vi "PLC_Trigger_Gen.vi"(5 "0_Stop":bool, 6 "Product Code":string, 7 "Station Number":string, 10 "Trig":bool[](array[boolean]), 11 "Trig old":bool[](array[boolean])) -> (3 "State to Log":T1(array[cluster]))   [LabVIEW 2017]
panel:
  in  "Ack old":bool[](array[boolean])
  in  "Ack":bool[](array[boolean])
  in  "Station No":u32
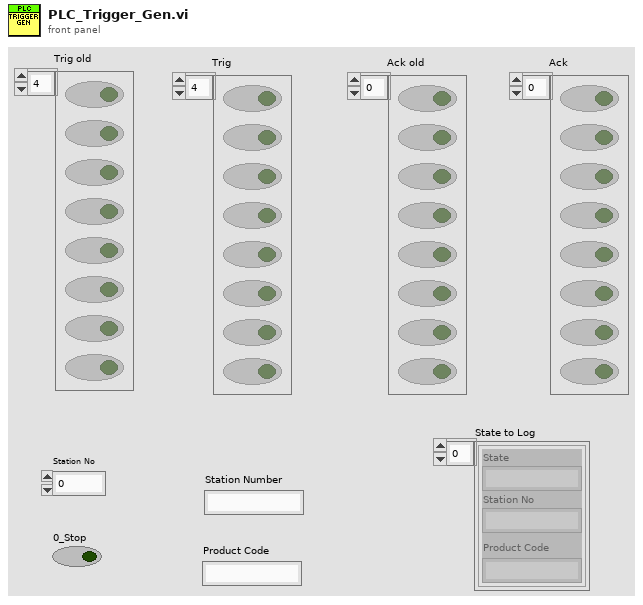
[diagram p1: front panel]
types:
  T1 = cluster{"State":string, "Station No":string, "Product Code":string}[]
  T2 = cluster{"State":string, "Station No":string, "Product Code":string}
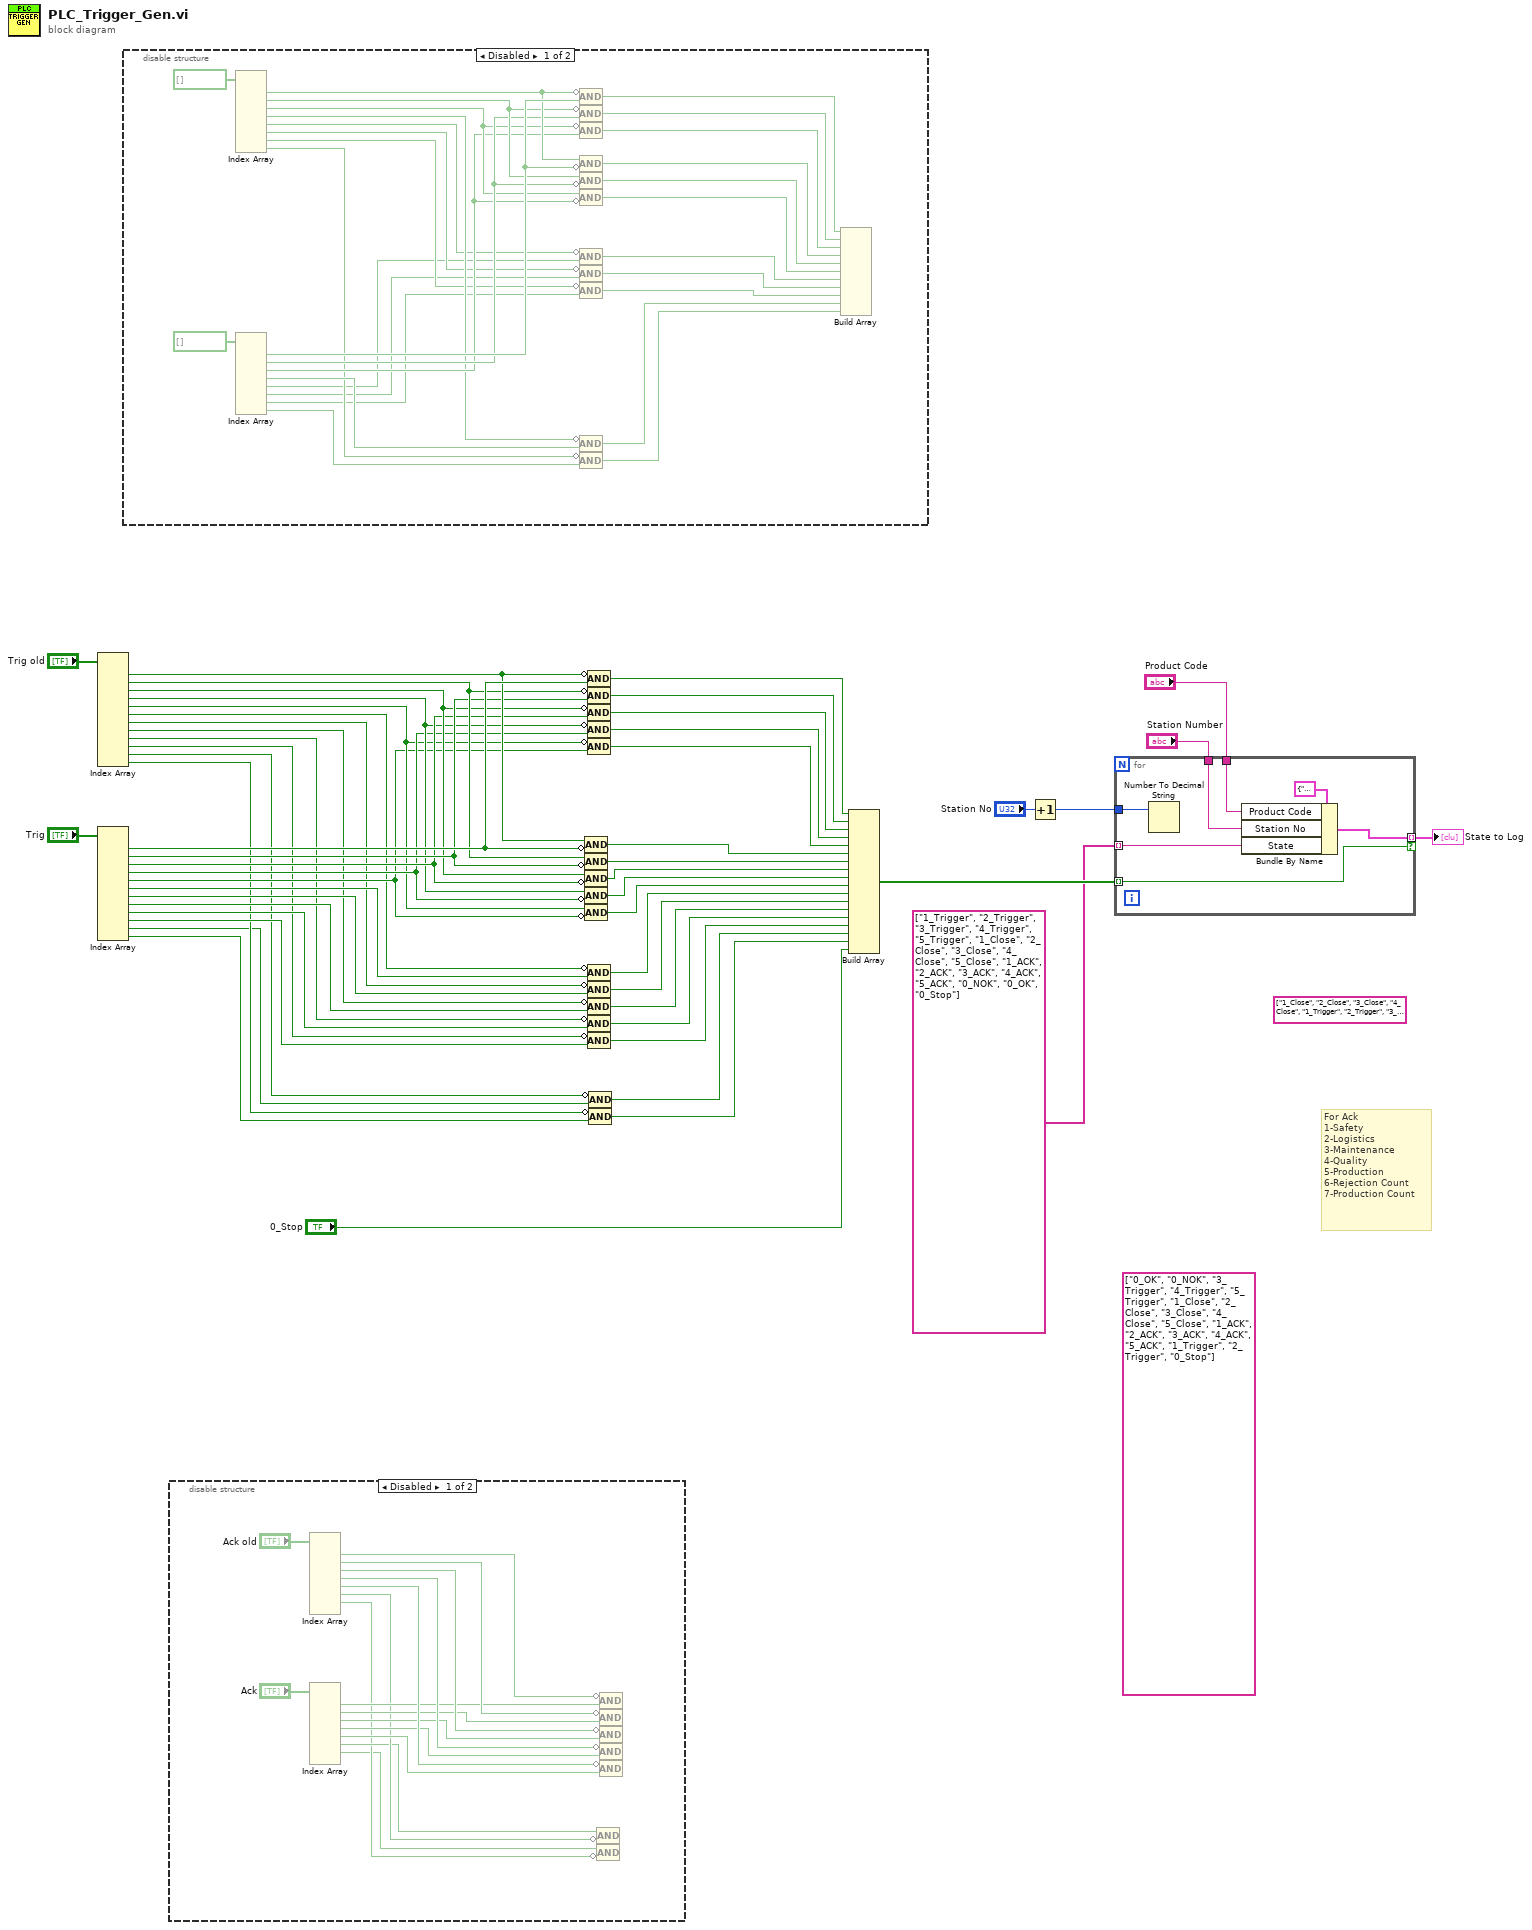
[diagram p0: block diagram]
diagram:
  (unwired) string[] ["1_Close", "2_Close", "3_Close", "4_Close", "1_Trigger", "2_Trigger", "3_Trigger", "4_Trigger", "1_ACK", "2_ACK", "3_ACK", "4_ACK", "0_Stop", "0_OK", "0_NOK"]
  (unwired) string[] ["0_OK", "0_NOK", "3_Trigger", "4_Trigger", "5_Trigger", "1_Close", "2_Close", "3_Close", "4_Close", "5_Close", "1_ACK", "2_ACK", "3_ACK", "4_ACK", "5_ACK", "1_Trigger", "2_Trigger", "0_Stop"]
  # "For Ack\n1-Safety\n2-Logistics\n3-Maintenance\n4-Quality\n5-Production\n6-Rejection Count\n7-Production Count"
  n1 = Index Array(array="Trig old") -> (element #1=w48:bool, element #2=w47:bool, element #3=w45:bool, element #4=w43:bool, element #5=w41:bool, element #6=w22:bool, element #7=w20:bool, element #8=w18:bool, element #9=w16:bool, element #10=w14:bool, element #11=w12:bool, element #12=w11:bool)  [unwired: 12 in]
  n2 = Index Array(array="Trig") -> (element #1=w49:bool, element #2=w46:bool, element #3=w44:bool, element #4=w42:bool, element #5=w40:bool, element #6=w21:bool, element #7=w19:bool, element #8=w17:bool, element #9=w15:bool, element #10=w13:bool, element #11=w10:bool, element #12=w2:bool)  [unwired: 12 in]
  n3 = disable-structure shown="Disabled" {
    frame Disabled {
      n4 = Index Array(array=bool[] []) -> (element #1=w79:bool, element #2=w78:bool, element #3=w76:bool, element #4=w74:bool, element #5=w64:bool, element #6=w63:bool, element #7=w62:bool, element #8=w69:bool)  [unwired: 8 in]
      n5 = Index Array(array=bool[] []) -> (element #1=w80:bool, element #2=w77:bool, element #3=w75:bool, element #4=w73:bool, element #5=w61:bool, element #6=w60:bool, element #7=w59:bool, element #8=w68:bool)  [unwired: 8 in]
      n6 = Compound Arithmetic op=AND(invert w79, w80) -> (w72:bool)
      n7 = Compound Arithmetic op=AND(invert w78, w77) -> (w71:bool)
      n8 = Compound Arithmetic op=AND(invert w76, w75) -> (w70:bool)
      n9 = Compound Arithmetic op=AND(w79, invert w80) -> (w67:bool)
      n10 = Compound Arithmetic op=AND(w78, invert w77) -> (w66:bool)
      n11 = Compound Arithmetic op=AND(w76, invert w75) -> (w65:bool)
      n12 = Compound Arithmetic op=AND(invert w64, w61) -> (w58:bool)
      n13 = Compound Arithmetic op=AND(invert w63, w60) -> (w56:bool)
      n14 = Compound Arithmetic op=AND(invert w62, w59) -> (w57:bool)
      n15 = Compound Arithmetic op=AND(invert w74, w73) -> (w55:bool)
      n16 = Compound Arithmetic op=AND(invert w69, w68) -> (w54:bool)
      n17 = Build Array(w72, w71, w70, w67, w66, w65, w58, w56, w57, w55, w54) -> ()  [unwired: 1 out]
    }
    frame Enabled {
    }
  }
  n18 = disable-structure shown="Disabled" {
    frame Disabled {
      n19 = Index Array(array="Ack old") -> (element #1=w88:bool, element #2=w89:bool, element #3=w91:bool, element #4=w93:bool, element #5=w95:bool, element #6=w84:bool, element #7=w82:bool)  [unwired: 8 in, 1 out]
      n20 = Index Array(array="Ack") -> (element #1=w87:bool, element #2=w90:bool, element #3=w92:bool, element #4=w94:bool, element #5=w96:bool, element #6=w83:bool, element #7=w81:bool)  [unwired: 8 in, 1 out]
      n21 = Compound Arithmetic op=AND(w83, invert w84) -> ()  [unwired: 1 out]
      n22 = Compound Arithmetic op=AND(w81, invert w82) -> ()  [unwired: 1 out]
      n23 = Compound Arithmetic op=AND(invert w88, w87) -> ()  [unwired: 1 out]
      n24 = Compound Arithmetic op=AND(invert w89, w90) -> ()  [unwired: 1 out]
      n25 = Compound Arithmetic op=AND(invert w91, w92) -> ()  [unwired: 1 out]
      n26 = Compound Arithmetic op=AND(invert w93, w94) -> ()  [unwired: 1 out]
      n27 = Compound Arithmetic op=AND(invert w95, w96) -> ()  [unwired: 1 out]
    }
    frame Enabled {
    }
  }
  n28 = Compound Arithmetic op=AND(w48, invert w49) -> (w34:bool)
  n29 = Compound Arithmetic op=AND(w47, invert w46) -> (w33:bool)
  n30 = Compound Arithmetic op=AND(w45, invert w44) -> (w32:bool)
  n31 = Compound Arithmetic op=AND(w43, invert w42) -> (w31:bool)
  n32 = Compound Arithmetic op=AND(w41, invert w40) -> (w30:bool)
  n33 = Compound Arithmetic op=AND(invert w48, w49) -> (w39:bool)
  n34 = Compound Arithmetic op=AND(invert w47, w46) -> (w38:bool)
  n35 = Compound Arithmetic op=AND(invert w45, w44) -> (w37:bool)
  n36 = Compound Arithmetic op=AND(invert w43, w42) -> (w36:bool)
  n37 = Compound Arithmetic op=AND(invert w41, w40) -> (w35:bool)
  n38 = Compound Arithmetic op=AND(invert w22, w21) -> (w9:bool)
  n39 = Compound Arithmetic op=AND(invert w20, w19) -> (w8:bool)
  n40 = Compound Arithmetic op=AND(invert w18, w17) -> (w7:bool)
  n41 = Compound Arithmetic op=AND(invert w16, w15) -> (w6:bool)
  n42 = Compound Arithmetic op=AND(invert w14, w13) -> (w5:bool)
  n43 = Compound Arithmetic op=AND(invert w12, w10) -> (w4:bool)
  n44 = Compound Arithmetic op=AND(invert w11, w2) -> (w3:bool)
  n45 = Build Array(w39, w38, w37, w36, w35, w34, w33, w32, w31, w30, w9, w8, w7, w6, w5, w4, w3, "0_Stop") -> (w28:bool[])
  n46 = Increment(x="Station No") -> (x+1=w29:u32)
  n47 = for {
    tunnel: w28 -> [w103] mode=indexing
    tunnel: string[] ["1_Trigger", "2_Trigger", "3_Trigger", "4_Trigger", "5_Trigger", "1_Close", "2_Close", "3_Close", "4_Close", "5_Close", "1_ACK", "2_ACK", "3_ACK", "4_ACK", "5_ACK", "0_NOK", "0_OK", "0_Stop"] -> [w101] mode=indexing
    tunnel: [w100] -> w26 mode=indexing if=w103
    tunnel: w29 -> [w99]
    tunnel: "Station Number" -> [w98]
    tunnel: "Product Code" -> [w97]
    n48 = Number To Decimal String(number=w99) -> ()  [unwired: 1 in, 1 out]
    n49 = Bundle By Name(cluster=T2 {"State"="", "Station No"="", "Product Code"=""}, "Product Code"=w97, "Station No"=w98, "State"=w101) -> (w100:T2)
  }
  "State to Log" <- w26
